vi "Main.vi"() -> ()   [LabVIEW 2020]
doc: "Cet exemple de projet Mesure continue est basé sur le modèle Gestionnaire de messages dans une file d'attente.\n\nLa boucle de gestion d'événements génère des messages en fonction des actions sur l'interface utilisateur.\n\nLa boucle de gestion de messages traite les messages générés par la boucle de gestion d'événements ou par d'autres messages. Il y a aussi des sous-VIs de boucle de gestion de messages d'acquisition et d'enregistrement, ainsi qu'une boucle de mise à jour du graphe déroulant."
uses:
  Settings/Settings.ctl
  Acquisition/Hardware Configuration.ctl
  Acquisition/Signal Type.ctl
  Logging/Logging Configuration.ctl
  controls/UI Data.ctl
  controls/UI State.ctl
  <vilib>/Waveform/WDTOps.llb/WDT Index Channel DBL.vi
  support/Message Queue/Enqueue Message (Single).vi
  support/Message Queue/Enqueue Message (Array).vi
  <vilib>/Utility/error.llb/Error Cluster From Error Code.vi
  <vilib>/ErrorRing/Error Ring.xnode
  Acquisition/Acquisition.lvlib
  Logging/Logging.lvlib
  Settings/Settings.lvlib
  support/User Event - Stop/User Event - Stop.lvlib
  support/Message Queue/Message Queue.lvlib
  Settings/Settings Dialog.vi
panel:
  in  "Panneaux":T1(tab)
  in  "Moyennage sélectionneur":bool
  in  "Choix moyennage":dbl
  in  "Mode longueur d'onde":bool=TRUE
  in  "Sélectionneur de longueur d'onde":dbl=500.0 min=500.0 max=2500.0 step=1.0
  in  "Longueur d'onde":bool
  out "Données":waveform(dbl)[](graph)
  out "État":string
  in  "Quitter":bool
  in  "Arrêter":bool
  in  "Démarrer":bool
  in  "Paramètres":bool
  out "Tableau 2":dbl[](array[numeric])
  # "MAPA Tech"
  # "Automatique"
  # "Manuel"
  # "MAPA Tech"
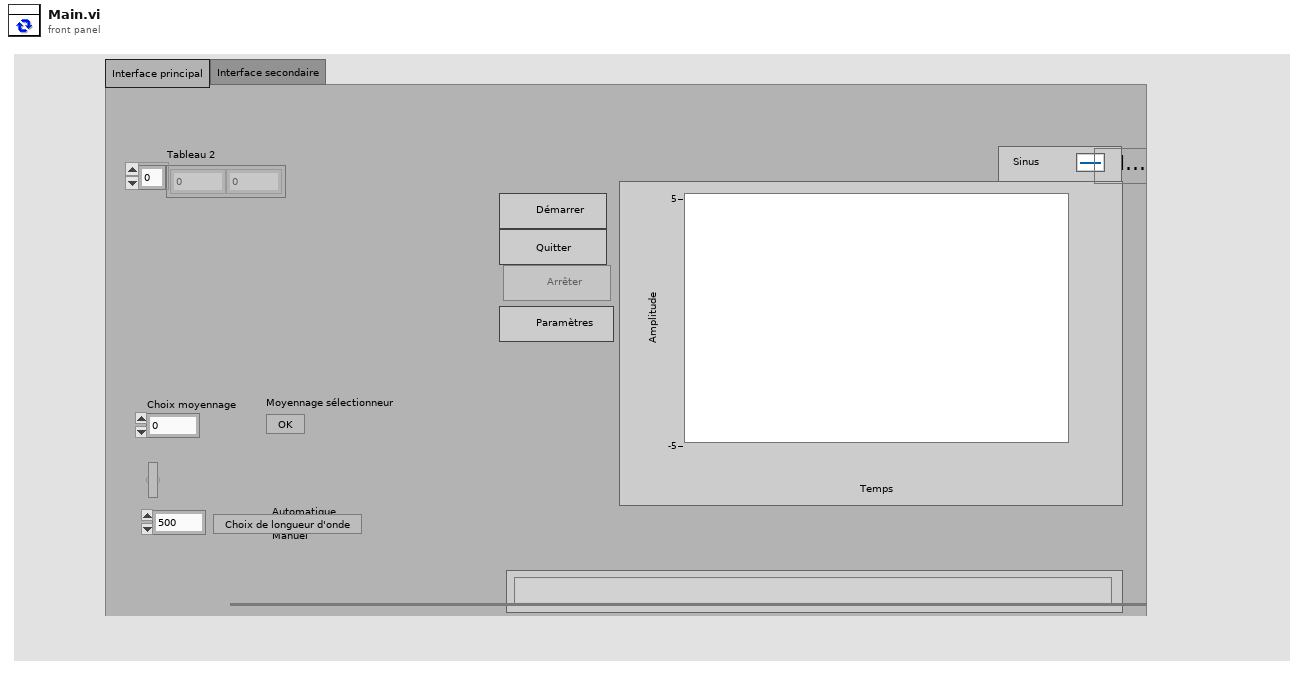
[diagram p1: front panel]
types:
  T1 = enum32{"Interface principal", "Interface secondaire"}
  T2 = typedef "UI State.ctl" = enum16{"Idle", "Acquiring and Logging", "Waiting for Exit", "Waiting for Exit (Acq Stopped)", "Waiting for Exit (Log Stopped)", "Waiting for Stop", "Waiting for Stop (Acq Stopped)", "Waiting for Stop (Log Stopped)"}
  T3 = typedef "UI Data.ctl" = cluster{"Réf. de Démarrer":refnum<vi>, "Réf. d'Arrêter":refnum<vi>, "Réf. de Paramètres":refnum<vi>, "Réf. de Quitter":refnum<vi>, "Réf. d'état":refnum<vi>, "Réf. de données":refnum<vi>, "Ref. longueur d'onde":refnum<vi>, "Ref. Choix mode longueur d'onde":refnum<vi>, "Ref. Moyennage sélectionneur":refnum<vi>}
  T4 = typedef "Settings.lvlib/Settings.ctl" = cluster{"Configuration du matériel":T5, "Configuration de l'enregistrement":T7, "Cluster test":cluster{"Numérique":dbl, "Numérique 2":dbl}}
  T5 = typedef "Acquisition.lvlib/Hardware Configuration.ctl" = cluster{"Refnum de matériel <À remplacer>":string, "Type de signal <À remplacer>":T6}
  T6 = typedef "Acquisition.lvlib/Signal Type.ctl" = enum16{"Sine Wave", "Square with Noise", "Signal triangulaire", "Simulation DAQ"}
  T7 = typedef "Logging.lvlib/Logging Configuration.ctl" = cluster{"Chemin de base du fichier journal":path, "Référence de fichier TDMS":refnum<k34>}
  T8 = cluster{"état":bool, "code":i32, "source":string}
  T9 = typedef "Message Queue.lvlib/All Message Queues.ctl" = cluster{"IU":refnum<queue>, "Acquisition":refnum<queue>, "Enregistrement":refnum<queue>}
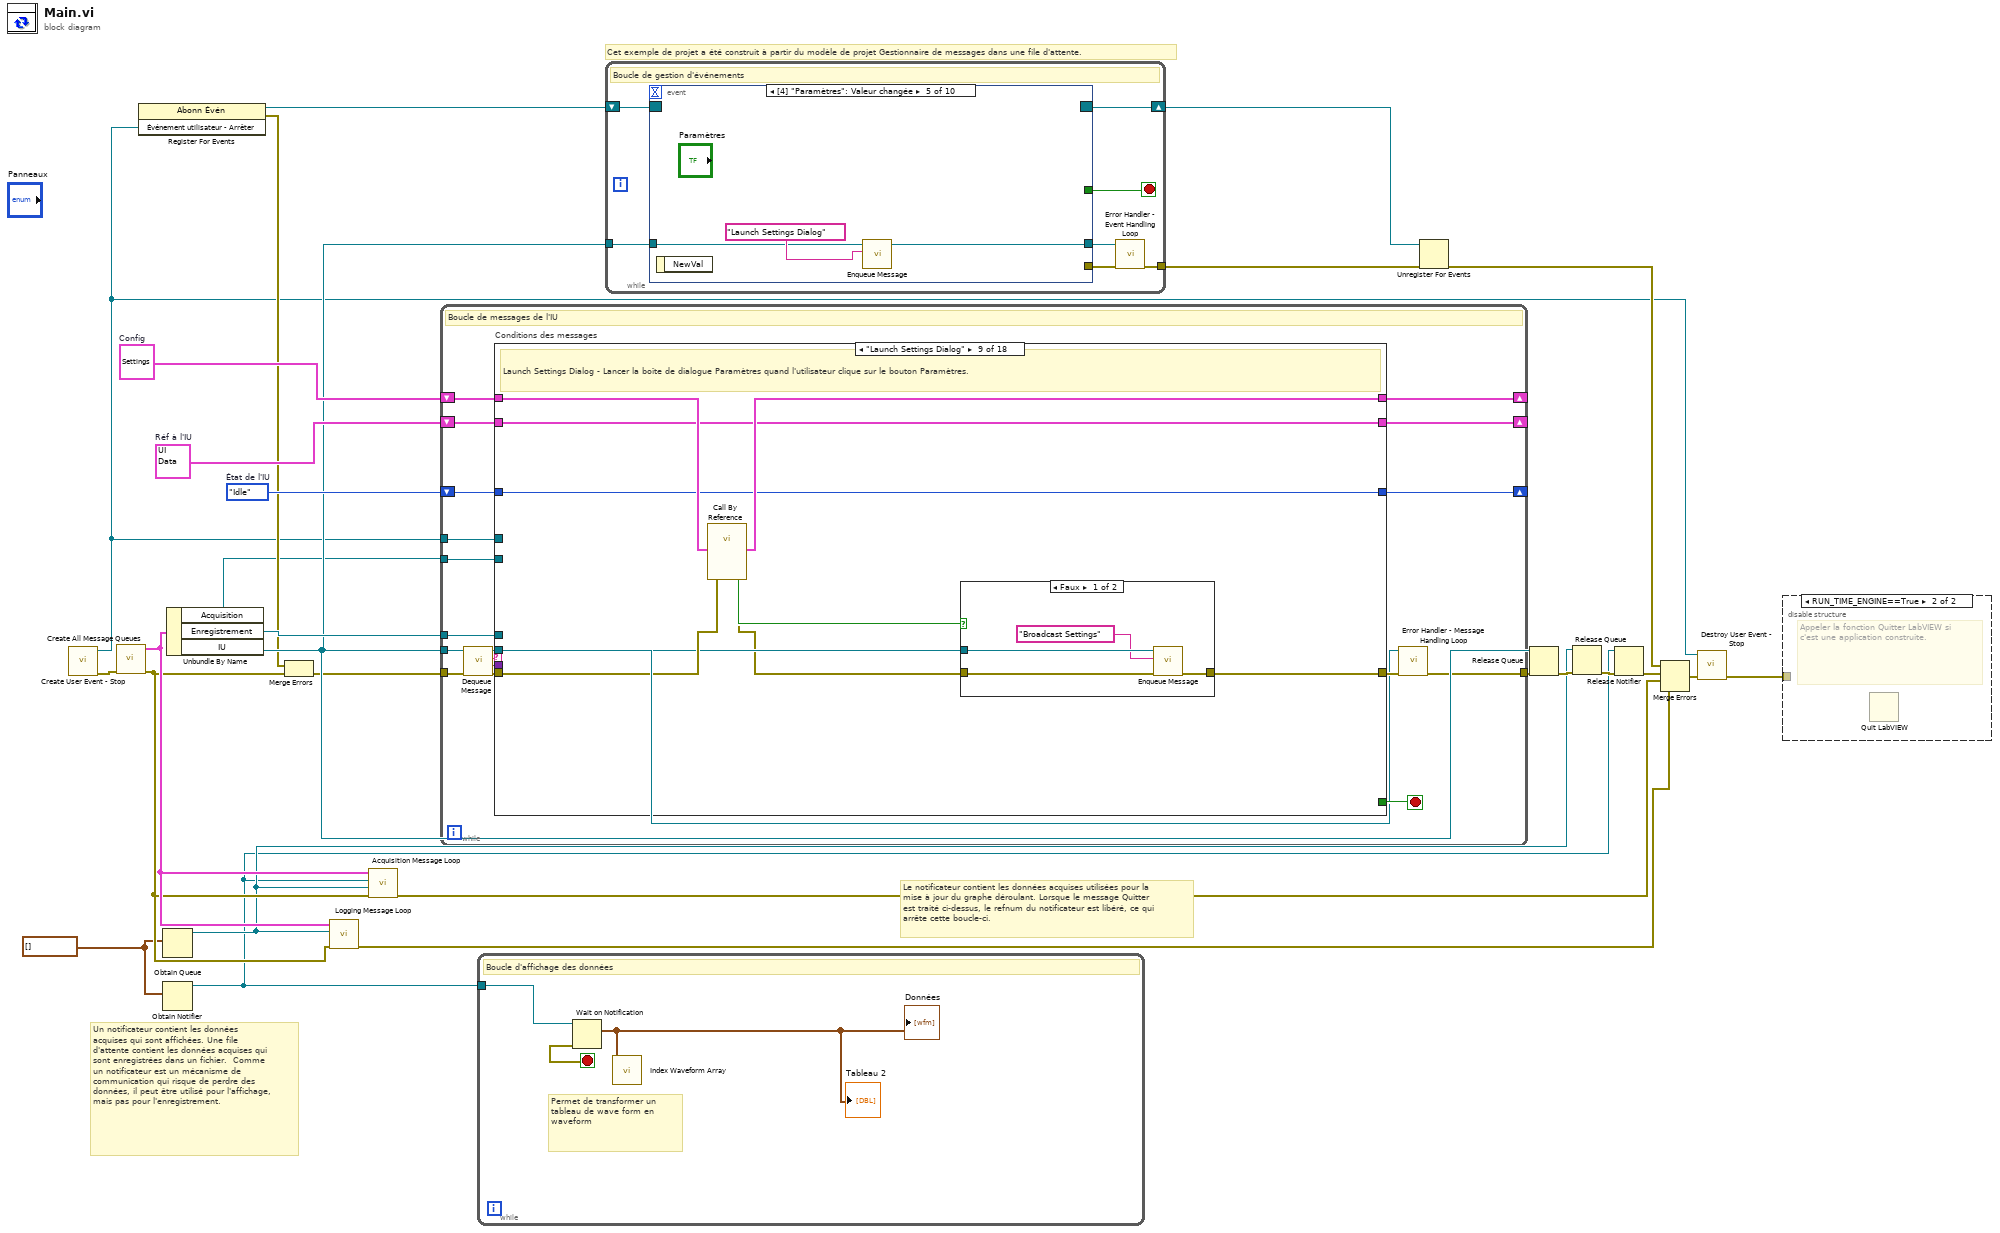
[diagram p0: block diagram]
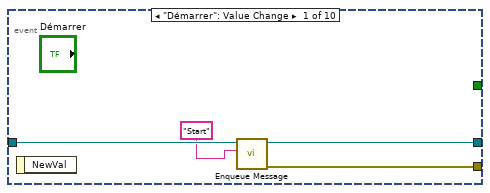
[diagram p3: hidden frame]
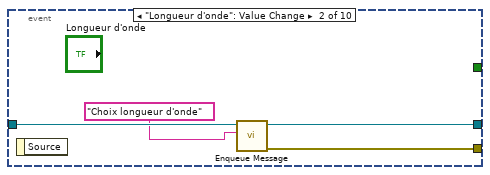
[diagram p4: hidden frame]
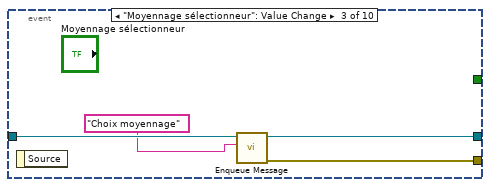
[diagram p5: hidden frame]
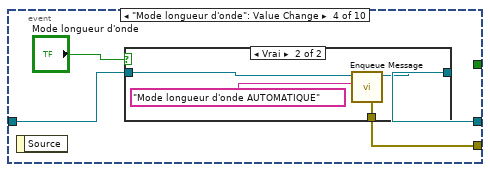
[diagram p6: hidden frame]
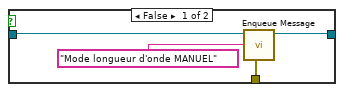
[diagram p7: hidden frame]
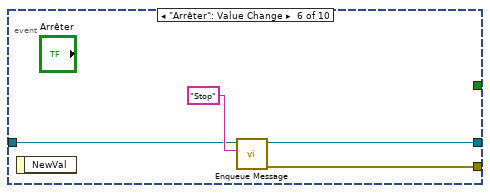
[diagram p8: hidden frame]
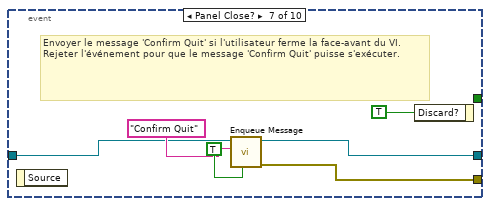
[diagram p9: hidden frame]
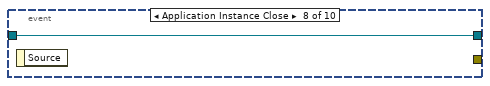
[diagram p10: hidden frame]
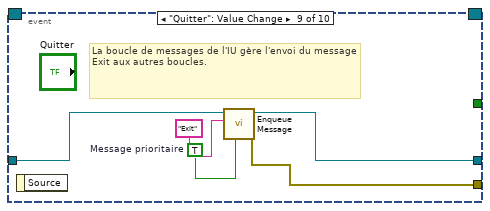
[diagram p11: hidden frame]
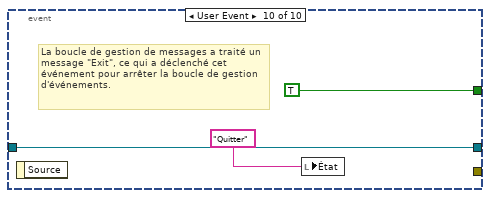
[diagram p12: hidden frame]
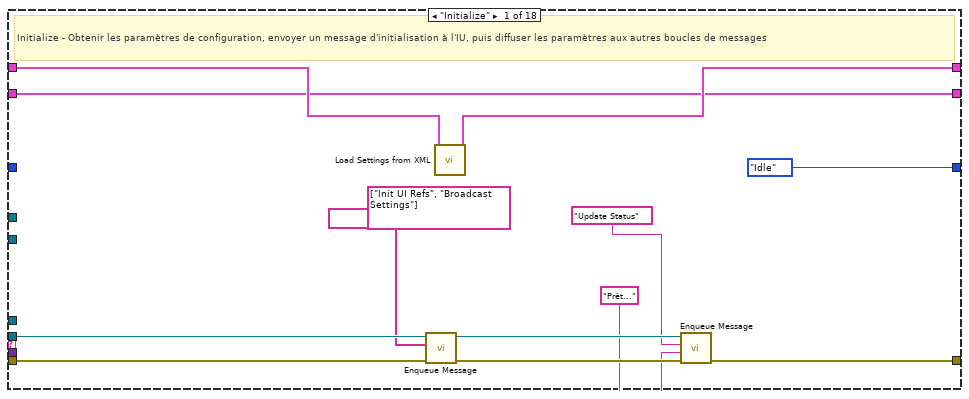
[diagram p13: hidden frame]
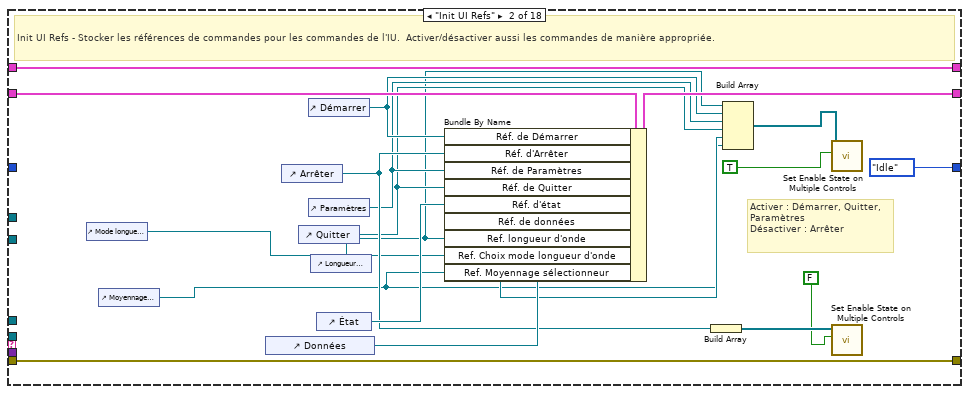
[diagram p14: hidden frame]
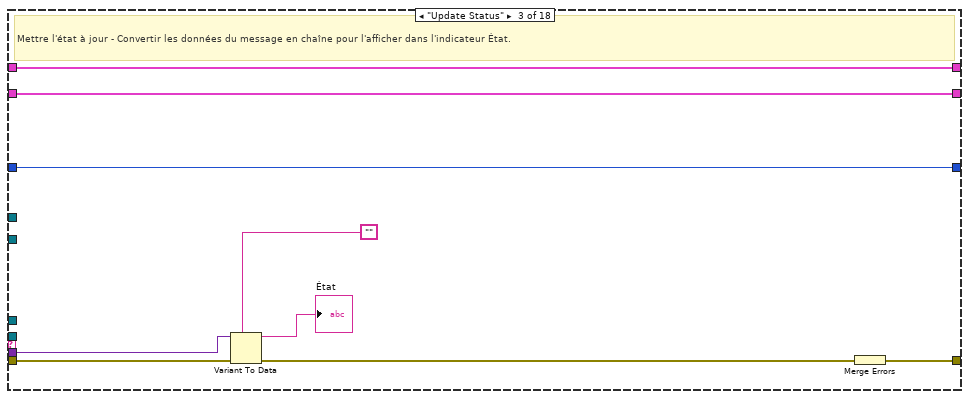
[diagram p15: hidden frame]
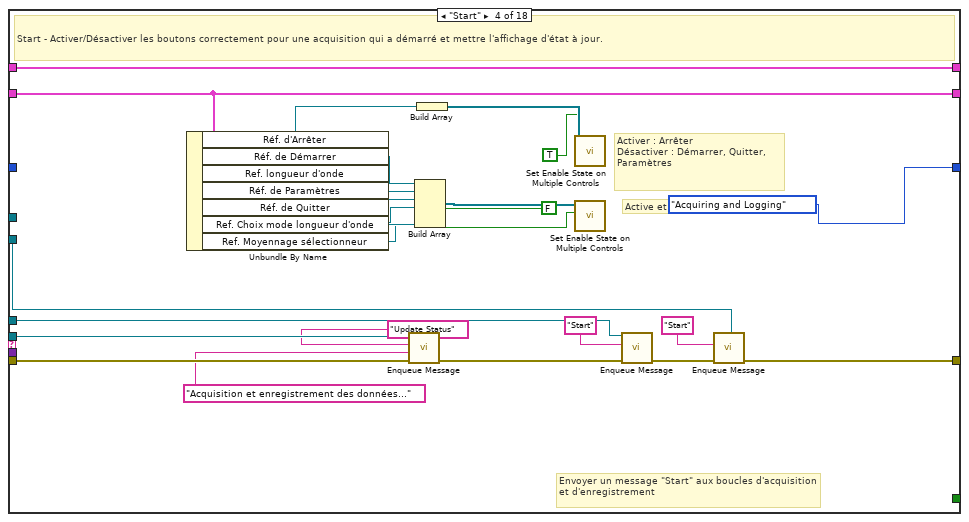
[diagram p16: hidden frame]
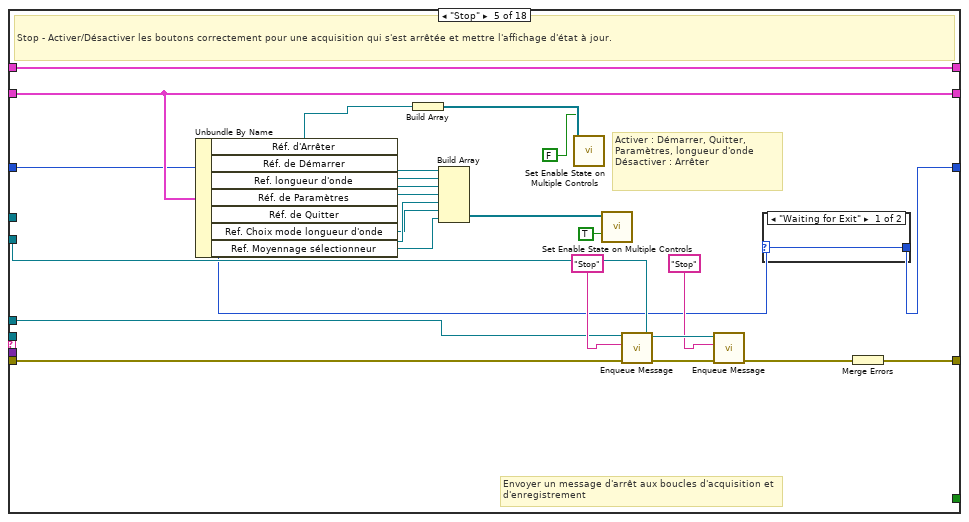
[diagram p17: hidden frame]
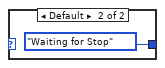
[diagram p18: hidden frame]
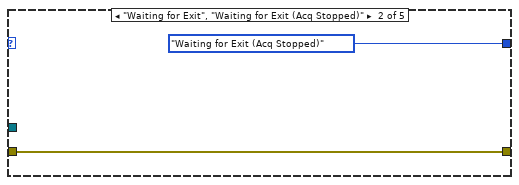
[diagram p20: hidden frame]
diagram:
  w15 = UI_State."Idle"  # État de l'IU
  w1 = waveform(dbl)[] []
  w17 = T3 {"Réf. de Démarrer"=refnum, "Réf. d'Arrêter"=refnum, "Réf. de Paramètres"=refnum, "Réf. de Quitter"=refnum, "Réf. d'état"=refnum, "Réf. de données"=refnum, "Ref. longueur d'onde"=refnum, "Ref. Choix mode longueur d'onde"=refnum, "Ref. Moyennage sélectionneur"=refnum}  # Réf à l'IU
  w20 = T4 {"Configuration du matériel"={"Refnum de matériel <À remplacer>"="", "Type de signal <À remplacer>"=enum."Simulation DAQ"}, "Configuration de l'enregistrement"={"Chemin de base du fichier journal"=path "", "Référence de fichier TDMS"=refnum}, "Cluster test"={"Numérique"=15.0, "Numérique 2"=0.0}}  # Config
  # "Cet exemple de projet a été construit à partir du modèle de projet Gestionnaire de messages dans une file d'attente."
  # "Un notificateur contient les données acquises qui sont affichées. Une file d'attente contient les données acquises qui sont enregistrées dans un fichier.  Comme un notificateur est un mécanisme de communication qui risque de perdre des données, il peut être utilisé pour l'affichage, mais pas pour l'enregistrement."
  # "Le notificateur contient les données acquises utilisées pour la mise à jour du graphe déroulant. Lorsque le message Quitter est traité ci-dessus, le refnum du notificateur est libéré, ce qui arrête cette boucle-ci."
  n1 = call "Create User Event - Stop.vi"() -> ("error out"=w24:T8, "Événement utilisateur - Arrêter"=w2:refnum<user-event>)  [unwired: 10 in]
  n2 = call "Create All Message Queues.vi"("error in (no error)"=w24) -> ("error out"=w21:T8, "Files d'attente de messages en sortie"=w23:T9)  [unwired: 9 in]
  n3 = register-events(w2) -> (reference out=w6:refnum<event-registration>, error out=w4:errorcluster)  [unwired: 2 in]
  n4 = Obtain Queue(element data type=w1) -> (queue out=w8:refnum<queue>)  [unwired: 4 in, 2 out]
  n5 = Obtain Notifier(notification data type=w1) -> (notifier out=w7:refnum<notifier>)  [unwired: 3 in, 2 out]
  n6 = Unbundle By Name(w23) -> ("Acquisition"=w3:refnum<queue>, "Enregistrement"=w16:refnum<queue>, "IU"=w13:refnum<queue>)
  n7 = Merge Errors(w4, w21) -> (w5:errorcluster)
  n8 = call "Logging Message Loop.vi"("error in (no error)"=w21, "File d'attente de données"=w8, "Files d'attente de messages"=w23) -> ("error out"=w22:T8)  [unwired: 8 in]
  n9 = call "Acquisition Message Loop.vi"("error in (no error)"=w21, "File d'attente de données"=w8, "Notificateur de données"=w7, "Files d'attente de messages"=w23) -> ("error out"=w25:T8)  [unwired: 7 in]
  n10 = while {
    tunnel: w13 -> [w39]
    tunnel: w2 -> [w44]
    shift-right: [w38] -> _
    shift-left: w20 -> [w37]
    shift-right: [w35] -> _
    shift-left: w17 -> [w36]
    tunnel: w3 -> [w34]
    tunnel: w16 -> [w33]
    shift-right: [w28] -> _
    shift-left: w15 -> [w29]
    tunnel: w5 -> [w43]
    tunnel: [w32] -> w27
    stop <- w45 stop-if-true
    # "Boucle de messages de l'IU"
    n11 = call "Dequeue Message.vi"("error in (no error)"=w43, "File d'attente de messages"=w39) -> ("error out"=w42:T8, "Données de message"=w40:variant, "Message"=w41:string, "File d'attente de message dup."=w30:refnum<queue>)  [unwired: 6 in]
    n12 = case "Conditions des messages" shown="\"Launch Settings Dialog\"" w41 {
      selector: w41 -> [_ _ _ _ _ _ _ _ _ _ _ _ _ _ _ _ _ w345]
      tunnel: w30 -> [w49 _ _ w109 _ w137 w162 _ w202 _ w223 _ _ w286 w306 w323 w340 _]
      tunnel: w42 -> [w48 w75 w83 w108 w131 w138 w163 w190 w204 w211 w222 w251 w268 w289 w309 w326 w343 _]
      tunnel: [w53 w75 w84 w93 w132 w135 w160 w196 w197 w214 w221 w261 w267 w288 w308 w325 w342 w344] -> w31
      tunnel: [_ _ _ _ _ _ _ _ _ _ _ TRUE _ _ _ _ _ _] -> w45
      tunnel: w40 -> [_ _ w82 _ _ _ _ _ _ w215 _ w249 _ _ _ _ _ _]
      tunnel: w44 -> [_ _ _ _ _ _ _ _ _ _ _ w262 _ _ _ _ _ _]
      tunnel: [w56 w74 w78 w107 w130 w141 w166 w194 w201 w219 w226 w260 w266 w287 w307 w324 w341 w348] -> w38
      tunnel: w37 -> [w57 w74 w78 w107 w130 w141 w166 w194 w205 w219 w226 w260 w266 w287 w307 w324 w341 w348]
      tunnel: w36 -> [w50 w73 w77 w104 w129 w140 w165 w188 w199 w218 w225 w259 w265 w277 w298 w317 w334 w347]
      tunnel: [w50 w70 w77 w104 w129 w140 w165 w188 w199 w218 w225 w259 w265 w277 w298 w317 w334 w347] -> w35
      tunnel: w34 -> [_ _ _ w92 w118 _ _ w187 _ _ _ w258 _ _ _ _ _ _]
      tunnel: w33 -> [_ _ _ w95 w121 _ _ w186 _ _ _ w257 _ _ _ _ _ _]
      tunnel: w29 -> [_ _ w76 _ w115 w139 w164 w185 w198 w213 w224 _ w264 _ _ _ _ w346]
      tunnel: [UI_State."Idle" ("UI State") UI_State."Idle" ("UI State") w76 UI_State."Acquiring and Logging" ("UI State") w116 w136 w161 w185 w198 w213 w220 UI_State."Idle" ("UI State") w264 UI_State."Acquiring and Logging" ("UI State") UI_State."Acquiring and Logging" ("UI State") UI_State."Acquiring and Logging" ("UI State") UI_State."Acquiring and Logging" ("UI State") w346] -> w28
      frame "Initialize" {
        # "Initialize - Obtenir les paramètres de configuration, envoyer un message d'initialisation à l'IU, puis diffuser les paramètres aux autres boucles de messages"
        n13 = call-poly "Enqueue Message.vi"("error in (no error)"=w48, "Tableau de messages"=string[] ["Init UI Refs", "Broadcast Settings"], "File d'attente de messages"=w49) -> ("error out"=w55:T8, "File d'attente de message dup."=w54:refnum<queue>)  [unwired: 7 in]
        n14 = call "Load Settings from XML.vi"("Paramètres en entrée"=w57) -> ("Paramètres en sortie"=w56:T4)  [unwired: 9 in, 1 out]
        n15 = call-poly "Enqueue Message.vi"("error in (no error)"=w55, "Données de message"="Prêt..." ("Ready..."), "Message"="Update Status", "File d'attente de messages"=w54) -> ("error out"=w53:T8)  [unwired: 6 in, 1 out]
      }
      frame "Init UI Refs" {
        # "Activer : Démarrer, Quitter, Paramètres\nDésactiver : Arrêter"
        # "Init UI Refs - Stocker les références de commandes pour les commandes de l'IU.  Activer/désactiver aussi les commandes de manière appropriée."
        n16 = control-ref of="Mode longueur d'onde"() -> (w59:refnum<vi>)
        n17 = control-ref of="Moyennage sélectionneur"() -> (w58:refnum<vi>)
        n18 = control-ref of="Données"() -> (w71:refnum<vi>)
        n19 = control-ref of="Arrêter"() -> (w65:refnum<vi>)
        n20 = control-ref of="Quitter"() -> (w62:refnum<vi>)
        n21 = control-ref of="Démarrer"() -> (w64:refnum<vi>)
        n22 = control-ref of="Paramètres"() -> (w63:refnum<vi>)
        n23 = control-ref of="Longueur d'onde"() -> (w60:refnum<vi>)
        n24 = control-ref of="État"() -> (w72:refnum<vi>)
        n25 = Bundle By Name(cluster=w73, "Réf. de Démarrer"=w64, "Réf. d'Arrêter"=w65, "Réf. de Paramètres"=w63, "Réf. de Quitter"=w62, "Réf. d'état"=w72, "Réf. de données"=w71, "Ref. longueur d'onde"=w60, "Ref. Choix mode longueur d'onde"=w59, "Ref. Moyennage sélectionneur"=w58) -> (w70:T3)
        n26 = Build Array(w65) -> (w67:refnum<vi>[])
        n27 = Build Array(w60, w64, w63, w62, w59, w58) -> (w68:refnum<vi>[])
        n28 = call "Set Enable State on Multiple Controls.vi"("Activé ?"=TRUE ("Enable?"), "Commandes"=w68) -> ()  [unwired: 10 in]
        n29 = call "Set Enable State on Multiple Controls.vi"("Activé ?"=FALSE ("Enable?"), "Commandes"=w67) -> ()  [unwired: 10 in]
      }
      frame "Update Status" {
        # "Mettre l'état à jour - Convertir les données du message en chaîne pour l'afficher dans l'indicateur État."
        n30 = Variant To Data(error in=w83, type="" ("Empty String Constant"), Variant=w82) -> (data=→"État":string, error out=w80:errorcluster)
        n31 = Merge Errors(w80) -> (w84:errorcluster)
      }
      frame "Start" {
        # "Active et désactive les boutons!"
        # "Envoyer un message \"Start\" aux boucles d'acquisition et d'enregistrement"
        # "Activer : Arrêter\nDésactiver : Démarrer, Quitter, Paramètres"
        # "Start - Activer/Désactiver les boutons correctement pour une acquisition qui a démarré et mettre l'affichage d'état à jour."
        n32 = Unbundle By Name(w104) -> ("Réf. d'Arrêter"=w99:refnum<vi>, "Réf. de Démarrer"=w98:refnum<vi>, "Ref. longueur d'onde"=w89:refnum<vi>, "Réf. de Paramètres"=w88:refnum<vi>, "Réf. de Quitter"=w87:refnum<vi>, "Ref. Choix mode longueur d'onde"=w86:refnum<vi>, "Ref. Moyennage sélectionneur"=w85:refnum<vi>)
        n33 = call-poly "Enqueue Message.vi"("error in (no error)"=w108, "Données de message"="Acquisition et enregistrement des données..." ("Acquiring and Logging..."), "Message"="Update Status", "File d'attente de messages"=w109) -> ("error out"=w97:T8)  [unwired: 6 in, 1 out]
        n34 = Build Array(w98, w89, w88, w87, w86, w85) -> (w102:refnum<vi>[])
        n35 = Build Array(w99) -> (w101:refnum<vi>[])
        n36 = call "Set Enable State on Multiple Controls.vi"("Activé ?"=TRUE ("Enable?"), "Commandes"=w101) -> ()  [unwired: 10 in]
        n37 = call "Set Enable State on Multiple Controls.vi"("Activé ?"=FALSE ("Enable?"), "Commandes"=w102) -> ()  [unwired: 10 in]
        n38 = call-poly "Enqueue Message.vi"("error in (no error)"=w97, "Message"="Start", "File d'attente de messages"=w95) -> ("error out"=w94:T8)  [unwired: 7 in, 1 out]
        n39 = call-poly "Enqueue Message.vi"("error in (no error)"=w94, "Message"="Start", "File d'attente de messages"=w92) -> ("error out"=w93:T8)  [unwired: 7 in, 1 out]
      }
      frame "Stop" {
        # "Envoyer un message d'arrêt aux boucles d'acquisition et d'enregistrement"
        # "Activer : Démarrer, Quitter, Paramètres, longueur d'onde\nDésactiver : Arrêter"
        # "Stop - Activer/Désactiver les boutons correctement pour une acquisition qui s'est arrêtée et mettre l'affichage d'état à jour."
        n40 = Unbundle By Name(w129) -> ("Réf. d'Arrêter"=w124:refnum<vi>, "Réf. de Démarrer"=w123:refnum<vi>, "Ref. longueur d'onde"=w114:refnum<vi>, "Réf. de Paramètres"=w113:refnum<vi>, "Réf. de Quitter"=w112:refnum<vi>, "Ref. Choix mode longueur d'onde"=w111:refnum<vi>, "Ref. Moyennage sélectionneur"=w110:refnum<vi>)
        n41 = Build Array(w124) -> (w126:refnum<vi>[])
        n42 = Build Array(w114, w123, w114, w113, w112, w111, w110) -> (w127:refnum<vi>[])
        n43 = call "Set Enable State on Multiple Controls.vi"("Activé ?"=FALSE ("Enable?"), "Commandes"=w126) -> ()  [unwired: 10 in]
        n44 = call "Set Enable State on Multiple Controls.vi"("Activé ?"=TRUE ("Enable?"), "Commandes"=w127) -> ()  [unwired: 10 in]
        n45 = call-poly "Enqueue Message.vi"("error in (no error)"=w131, "Message"="Stop", "File d'attente de messages"=w121) -> ("error out"=w120:T8)  [unwired: 7 in, 1 out]
        n46 = call-poly "Enqueue Message.vi"("error in (no error)"=w120, "Message"="Stop", "File d'attente de messages"=w118) -> ("error out"=w119:T8)  [unwired: 7 in, 1 out]
        n47 = case shown="\"Waiting for Exit\"" w115 {
          selector: w115 -> [w133 _]
          tunnel: [w133 UI_State."Waiting for Stop" ("UI State")] -> w116
          frame "Waiting for Exit" {
          }
          frame Default {
          }
        }
        n48 = Merge Errors(w119) -> (w132:errorcluster)
      }
      frame "Acquisition Stopped" {
        # "Logique déterminant quelle action entreprendre quand l'acquisition s'est arrêtée."
        n49 = case shown="Par défaut" w139 {
          selector: w139 -> [w143 _ _ _ _]
          tunnel: w138 -> [w142 w145 w147 w153 w159]
          tunnel: w137 -> [_ _ _ w151 w156]
          tunnel: [w143 UI_State."Waiting for Exit (Acq Stopped)" ("UI State") UI_State."Waiting for Stop (Acq Stopped)" ("UI State") UI_State."Idle" ("UI State") UI_State."Idle" ("UI State")] -> w136
          tunnel: [w142 w145 w147 w152 w157] -> w135
          frame Default {
          }
          frame "Waiting for Exit", "Waiting for Exit (Acq Stopped)" {
          }
          frame "Waiting for Stop", "Waiting for Stop (Acq Stopped)" {
          }
          frame "Waiting for Exit (Log Stopped)" {
            # "Si nous attendons pour quitter et que l'enregistrement s'est déjà arrêté, le message \"Acquisition Stopped\" indique qu'il est temps de quitter."
            n50 = call-poly "Enqueue Message.vi"("Message prioritaire ? (F)"=TRUE ("Priority Message? (F)"), "error in (no error)"=w153, "Message"="Exit", "File d'attente de messages"=w151) -> ("error out"=w152:T8)  [unwired: 6 in, 1 out]
          }
          frame "Waiting for Stop (Log Stopped)" {
            # "Si nous attendons pour arrêter et que l'enregistrement s'est déjà arrêté, le message \"Acquisition Stopped\" indique qu'il est temps d'arrêter."
            n51 = call-poly "Enqueue Message.vi"("error in (no error)"=w159, "Données de message"="Prêt..." ("Ready..."), "Message"="Update Status", "File d'attente de messages"=w156) -> ("error out"=w157:T8)  [unwired: 6 in, 1 out]
          }
        }
      }
      frame "Logging Stopped" {
        # "Logique déterminant quelle action entreprendre quand l'enregistrement s'est arrêté."
        n52 = case shown="\"Waiting for Stop (Acq Stopped)\"" w164 {
          selector: w164 -> [w168 _ _ _ _]
          tunnel: w163 -> [w167 w170 w172 w178 w181]
          tunnel: w162 -> [_ _ _ w176 w180]
          tunnel: [w168 UI_State."Waiting for Exit (Log Stopped)" ("UI State") UI_State."Waiting for Stop (Log Stopped)" ("UI State") UI_State."Idle" ("UI State") UI_State."Idle" ("UI State")] -> w161
          tunnel: [w167 w170 w172 w177 w179] -> w160
          frame Default {
          }
          frame "Waiting for Exit", "Waiting for Exit (Log Stopped)" {
          }
          frame "Waiting for Stop", "Waiting for Stop (Log Stopped)" {
          }
          frame "Waiting for Exit (Acq Stopped)" {
            # "Si nous attendons pour quitter et que l'acquisition s'est déjà arrêtée, le message \"Logging Stopped\" indique qu'il est temps de quitter."
            n53 = call-poly "Enqueue Message.vi"("Message prioritaire ? (F)"=TRUE ("Priority Message? (F)"), "error in (no error)"=w178, "Message"="Exit", "File d'attente de messages"=w176) -> ("error out"=w177:T8)  [unwired: 6 in, 1 out]
          }
          frame "Waiting for Stop (Acq Stopped)" {
            # "Si nous attendons pour arrêter et que l'acquisition s'est déjà arrêtée, le message \"Logging Stopped\" indique qu'il est temps d'arrêter."
            n54 = call-poly "Enqueue Message.vi"("error in (no error)"=w181, "Données de message"="Prêt..." ("Ready..."), "Message"="Update Status", "File d'attente de messages"=w180) -> ("error out"=w179:T8)  [unwired: 6 in, 1 out]
          }
        }
      }
      frame "Broadcast settings" {
        w189 = "Update Settings" ("Message")
        # "Broadcast settings - Envoyer le message 'Update Settings' aux boucles de messages d'enregistrement et d'acquisition."
        n55 = Unbundle By Name(w194) -> ("Configuration du matériel"=w193:T5, "Configuration de l'enregistrement"=w192:T7)
        n56 = call-poly "Enqueue Message.vi"("Données de message"=w193, "Message"=w189, "File d'attente de messages"=w187) -> ("error out"=w195:T8)  [unwired: 7 in, 1 out]
        n57 = call-poly "Enqueue Message.vi"("error in (no error)"=w195, "Données de message"=w192, "Message"=w189, "File d'attente de messages"=w186) -> ("error out"=w191:T8)  [unwired: 6 in, 1 out]
        n58 = Merge Errors(w191, w190) -> (w196:errorcluster)
      }
      frame "Launch Settings Dialog" {
        # "Launch Settings Dialog - Lancer la boîte de dialogue Paramètres quand l'utilisateur clique sur le bouton Paramètres."
        n59 = call-by-ref "?"("error in (no error)"=w204, "Paramètres en entrée"=w205) -> ("error out"=w200:T8, "Annulation ?"=w203:bool, "Paramètres en sortie"=w201:T4)  [unwired: 8 in, 3 out]
        n60 = case shown="Faux" w203 {
          tunnel: w202 -> [w209 _]
          tunnel: w200 -> [w208 w210]
          tunnel: [w207 w210] -> w197
          frame False {
            n61 = call-poly "Enqueue Message.vi"("error in (no error)"=w208, "Message"="Broadcast Settings", "File d'attente de messages"=w209) -> ("error out"=w207:T8)  [unwired: 7 in, 1 out]
          }
          frame True {
          }
        }
      }
      frame "Error" {
        # "Error - Afficher une boîte de dialogue d'erreur. Ce message est envoyé par les VIs \"Error Handler\" à la fin de l'exécution de chaque boucle de cette application."
        n62 = Variant To Data(error in=w211, type=errorcluster {"status"=FALSE, "code"=0, "source"=""} ("error constant"), Variant=w215) -> (data=w212:errorcluster, error out=w216:errorcluster)
        n63 = call <vilib>:"Simple Error Handler.vi"("error in (no error)"=w212) -> ()  [unwired: 4 in, 5 out]
        n64 = Merge Errors(w216) -> (w214:errorcluster)
      }
      frame "Confirm Quit" {
        # "Confirm Quit - Message qui confirme si l'utilisateur voulait vraiment quitter l'application."
        n65 = case shown="\"Acquiring and Logging\"" w224 {
          tunnel: w223 -> [w232 w236]
          tunnel: w222 -> [w231 w235]
          tunnel: [w230 w234] -> w221
          tunnel: [UI_State."Idle" ("UI State") w233] -> w220
          frame Default {
            # "Si 'Confirm Quit' survient alors que le système est inactif, le message de confirmation est inutile."
            n66 = call-poly "Enqueue Message.vi"("Message prioritaire ? (F)"=TRUE ("Priority Message? (F)"), "error in (no error)"=w231, "Message"="Exit", "File d'attente de messages"=w232) -> ("error out"=w230:T8)  [unwired: 6 in, 1 out]
          }
          frame "Acquiring and Logging" {
            n67 = Two Button Dialog(message="Voulez-vous vraiment quitter en cours d'acquisition ?" ("Confirm Quit Message"), 1:"Non" ("No"), 2:"Oui" ("Yes")) -> (T button?=w237:bool)
            n68 = case shown="Vrai" w237 {
              tunnel: w236 -> [_ w246]
              tunnel: w235 -> [w242 w247]
              tunnel: [w242 w245] -> w234
              tunnel: [UI_State."Acquiring and Logging" ("UI State") UI_State."Waiting for Exit" ("UI State")] -> w233
              frame False {
                # "L'utilisateur ne voulait pas quitter."
              }
              frame True {
                n69 = call-poly "Enqueue Message.vi"("error in (no error)"=w247, "Message"="Stop", "File d'attente de messages"=w246) -> ("error out"=w245:T8)  [unwired: 7 in, 1 out]
              }
            }
          }
        }
      }
      frame "Exit" {
        w253 = TRUE ("Priority Message? (F)")
        w254 = "Exit" ("Message")
        # "Afficher une boîte de dialogue d'erreur si 'Exit' a été appelé suite à une erreur."
        # "Arrêter le VI"
        # "Exit - Envoyer des messages Exit aux boucles d'acquisition et d'enregistrerment, et déclencher l'événement utilisateur pour arrêter la boucle de gestion d'événements."
        n70 = Variant To Data(type=errorcluster {"status"=FALSE, "code"=0, "source"=""} ("error constant"), Variant=w249) -> (data=w248:errorcluster)  [unwired: 1 in, 1 out]
        n71 = call <vilib>:"Simple Error Handler.vi"("error in (no error)"=w248) -> ()  [unwired: 4 in, 5 out]
        n72 = call-poly "Enqueue Message.vi"("Message prioritaire ? (F)"=w253, "error in (no error)"=w251, "Message"=w254, "File d'attente de messages"=w258) -> ("error out"=w255:T8)  [unwired: 6 in, 1 out]
        n73 = call-poly "Enqueue Message.vi"("Message prioritaire ? (F)"=w253, "error in (no error)"=w255, "Message"=w254, "File d'attente de messages"=w257) -> ("error out"=w252:T8)  [unwired: 6 in, 1 out]
        n74 = call "Fire User Event - Stop.vi"("error in (no error)"=w252, "Événement utilisateur - Arrêt"=w262) -> ("error out"=w261:T8)  [unwired: 9 in]
      }
      frame "---Copy This Frame---" {
        # "Dupliquez cette étape pour créer de nouveaux messages.  Changez ce commentaire dans l'étape dupliquée pour décrire ce message."
        n75 = Merge Errors(w268) -> (w267:errorcluster)
      }
      frame "Choix longueur d'onde" {
        # "Activer : \nDésactiver :"
        # "Affiche la longueur d'onde en live.\nComment je fais pour limiter le range\ncomment je fais pour afficher pas en live\ngestion d'erreur?"
        # "Dupliquez cette étape pour créer de nouveaux messages.  Changez ce commentaire dans l'étape dupliquée pour décrire ce message."
        n76 = Unbundle By Name(w277) -> ("Ref. longueur d'onde"=w274:refnum<vi>, "Réf. d'Arrêter"=w272:refnum<vi>, "Réf. de Démarrer"=w271:refnum<vi>, "Réf. de Quitter"=w275:refnum<vi>, "Réf. de Paramètres"=w273:refnum<vi>)
        n77 = Build Array(w271, w275, w274, w273) -> (w279:refnum<vi>[])
        n78 = Build Array(w272) -> (w270:refnum<vi>[])
        n79 = call "Set Enable State on Multiple Controls.vi"("Activé ?"=TRUE ("Enable?"), "Commandes"=w279) -> ()  [unwired: 10 in]
        n80 = Number To Decimal String(number="Sélectionneur de longueur d'onde") -> (decimal integer string=w283:string)  [unwired: 1 in]
        n81 = Concatenate Strings ("Concaténer des chaînes")("La longueur d'onde sélectionné est de ", w283, " nm.") -> (w280:string)
        n82 = call "Set Enable State on Multiple Controls.vi"("Activé ?"=FALSE ("Enable?"), "Commandes"=w270) -> ()  [unwired: 10 in]
        n83 = call-poly "Enqueue Message.vi"("Données de message"=w280, "Message"="Update Status", "File d'attente de messages"=w286) -> ()  [unwired: 7 in, 2 out]
        n84 = Merge Errors(w289) -> (w288:errorcluster)
      }
      frame "Choix moyennage" {
        # "Activer : \nDésactiver :"
        # "Affiche la longueur d'onde en live.\nComment je fais pour limiter le range\ncomment je fais pour afficher pas en live\ngestion d'erreur?"
        # "Dupliquez cette étape pour créer de nouveaux messages.  Changez ce commentaire dans l'étape dupliquée pour décrire ce message."
        n85 = Unbundle By Name(w298) -> ("Réf. d'Arrêter"=w292:refnum<vi>, "Réf. de Démarrer"=w291:refnum<vi>, "Réf. de Quitter"=w296:refnum<vi>, "Réf. de Paramètres"=w290:refnum<vi>)
        n86 = Build Array(w291, w296, w290) -> (w300:refnum<vi>[])
        n87 = Build Array(w292) -> (w294:refnum<vi>[])
        n88 = call "Set Enable State on Multiple Controls.vi"("Activé ?"=TRUE ("Enable?"), "Commandes"=w300) -> ()  [unwired: 10 in]
        n89 = Number To Decimal String(number="Choix moyennage") -> (decimal integer string=w304:string)  [unwired: 1 in]
        n90 = call "Set Enable State on Multiple Controls.vi"("Activé ?"=FALSE ("Enable?"), "Commandes"=w294) -> ()  [unwired: 10 in]
        n91 = Concatenate Strings ("Concaténer des chaînes")("Le moyennage sélectionné est de ", w304, " Hz.") -> (w301:string)
        n92 = call-poly "Enqueue Message.vi"("Données de message"=w301, "Message"="Update Status", "File d'attente de messages"=w306) -> ()  [unwired: 7 in, 2 out]
        n93 = Merge Errors(w309) -> (w308:errorcluster)
      }
      frame "Mode longueur d'onde AUTOMATIQUE" {
        # "Activer : \nDésactiver :"
        # "Dupliquez cette étape pour créer de nouveaux messages.  Changez ce commentaire dans l'étape dupliquée pour décrire ce message."
        n94 = Unbundle By Name(w317) -> ("Ref. longueur d'onde"=w314:refnum<vi>, "Réf. d'Arrêter"=w312:refnum<vi>, "Réf. de Démarrer"=w311:refnum<vi>, "Réf. de Quitter"=w315:refnum<vi>, "Réf. de Paramètres"=w310:refnum<vi>)
        n95 = Build Array(w311, w315, w310) -> (w319:refnum<vi>[])
        n96 = Build Array(w312, w314) -> (w320:refnum<vi>[])
        n97 = call "Set Enable State on Multiple Controls.vi"("Activé ?"=TRUE ("Enable?"), "Commandes"=w319) -> ()  [unwired: 10 in]
        n98 = call "Set Enable State on Multiple Controls.vi"("Activé ?"=FALSE ("Enable?"), "Commandes"=w320) -> ()  [unwired: 10 in]
        n99 = call-poly "Enqueue Message.vi"("Données de message"="Le mode sélectionné pour la longueur d'onde est automatique.", "Message"="Update Status", "File d'attente de messages"=w323) -> ()  [unwired: 7 in, 2 out]
        n100 = Merge Errors(w326) -> (w325:errorcluster)
      }
      frame "Mode longueur d'onde MANUEL" {
        # "Activer : \nDésactiver :"
        # "Affiche la longueur d'onde en live.\nComment je fais pour limiter le range\ncomment je fais pour afficher pas en live\ngestion d'erreur?"
        # "Dupliquez cette étape pour créer de nouveaux messages.  Changez ce commentaire dans l'étape dupliquée pour décrire ce message."
        n101 = Unbundle By Name(w334) -> ("Ref. longueur d'onde"=w330:refnum<vi>, "Réf. d'Arrêter"=w329:refnum<vi>, "Réf. de Démarrer"=w328:refnum<vi>, "Réf. de Quitter"=w332:refnum<vi>, "Réf. de Paramètres"=w327:refnum<vi>)
        n102 = Build Array(w327, w328, w332, w330) -> (w336:refnum<vi>[])
        n103 = Build Array(w329) -> (w337:refnum<vi>[])
        n104 = call "Set Enable State on Multiple Controls.vi"("Activé ?"=TRUE ("Enable?"), "Commandes"=w336) -> ()  [unwired: 10 in]
        n105 = call "Set Enable State on Multiple Controls.vi"("Activé ?"=FALSE ("Enable?"), "Commandes"=w337) -> ()  [unwired: 10 in]
        n106 = call-poly "Enqueue Message.vi"("Données de message"="Le mode sélectionné pour la longueur d'onde est manuel.", "Message"="Update Status", "File d'attente de messages"=w340) -> ()  [unwired: 7 in, 2 out]
        n107 = Merge Errors(w343) -> (w342:errorcluster)
      }
      frame Default {
        # "La condition 'Par défaut' ne s'exécute que s'il y a un message qui n'est défini dans aucune des autres conditions.  Renvoyer une erreur de programmation."
        n108 = xnode ("Error Ring")("paramètre 0"=w345) -> ("sortie d'erreur"=w344:errorcluster)
      }
    }
    n109 = call "Error Handler - Message Handling Loop.vi"("error in (no error)"=w31, "File d'attente de messages"=w30) -> ("erreur en entrée dup."=w32:T8)  [unwired: 8 in, 1 out]
  }
  n110 = while "Data Display Loop" {
    tunnel: w7 -> [w357]
    stop <- w358 stop-if-true
    # "Permet de transformer un tableau de wave form en\nwaveform"
    # "Boucle d'affichage des données"
    n111 = Wait on Notification(notifier=w357) -> (notification=w356:waveform(dbl)[], error out=w358:errorcluster)  [unwired: 3 in, 2 out]
    "Données" <- w356
    "Tableau 2" <- w356
    n112 = call-poly <vilib>:"Index Waveform Array.vi"("waveform array"=w356) -> ()  [unwired: 9 in, 2 out]
  }
  n113 = while {
    tunnel: w13 -> [w364]
    tunnel: [w361] -> w26
    shift-right: [w363] -> w18
    shift-left: w6 -> [w365]
    stop <- w362 stop-if-true
    # "Boucle de gestion d'événements"
    n114 = event shown="[4] \"Paramètres\": Valeur changée" {
      selector: w365 -> [_ _ _ _ _ _ _ _ _ _]
      dyn-events: [_ _ _ _ _ _ _ _ _ _] -> w363
      timeout: _ -> [_ _ _ _ _ _ _ _ _ _]
      tunnel: [_ _ _ _ _ _ _ _ _ TRUE ("Discard?")] -> w362
      tunnel: w364 -> [w369 w373 w377 w380 w391 w395 w400 w403 w405 w409]
      tunnel: [w367 w371 w375 w379 _ w394 w398 _ w408 _] -> w360
      tunnel: [w366 w370 w374 w378 w390 w393 w399 w403 w404 w409] -> w359
      event "Démarrer": Value Change {
        n115 = event-data() -> ()  [unwired: 1 in, 1 out]
        n116 = call-poly "Enqueue Message.vi"("Message"="Start", "File d'attente de messages"=w369) -> ("error out"=w367:T8, "File d'attente de message dup."=w366:refnum<queue>)  [unwired: 8 in]
      }
      event "Longueur d'onde": Value Change {
        n117 = event-data() -> ()  [unwired: 1 in, 1 out]
        n118 = call-poly "Enqueue Message.vi"("Message"="Choix longueur d'onde", "File d'attente de messages"=w373) -> ("error out"=w371:T8, "File d'attente de message dup."=w370:refnum<queue>)  [unwired: 8 in]
      }
      event "Moyennage sélectionneur": Value Change {
        n119 = event-data() -> ()  [unwired: 1 in, 1 out]
        n120 = call-poly "Enqueue Message.vi"("Message"="Choix moyennage", "File d'attente de messages"=w377) -> ("error out"=w375:T8, "File d'attente de message dup."=w374:refnum<queue>)  [unwired: 8 in]
      }
      event "Mode longueur d'onde": Value Change {
        n121 = event-data() -> ()  [unwired: 1 in, 1 out]
        n122 = case shown="Vrai" "Mode longueur d'onde" {
          tunnel: w380 -> [w384 w389]
          tunnel: [w382 w388] -> w379
          tunnel: [w383 w387] -> w378
          frame False {
            n123 = call-poly "Enqueue Message.vi"("Message"="Mode longueur d'onde MANUEL", "File d'attente de messages"=w384) -> ("error out"=w382:T8, "File d'attente de message dup."=w383:refnum<queue>)  [unwired: 8 in]
          }
          frame True {
            n124 = call-poly "Enqueue Message.vi"("Message"="Mode longueur d'onde AUTOMATIQUE", "File d'attente de messages"=w389) -> ("error out"=w388:T8, "File d'attente de message dup."=w387:refnum<queue>)  [unwired: 8 in]
          }
        }
      }
      event "Paramètres": Value Change {
        n125 = event-data() -> ()  [unwired: 1 in, 1 out]
        n126 = call-poly "Enqueue Message.vi"("Message"="Launch Settings Dialog", "File d'attente de messages"=w391) -> ("File d'attente de message dup."=w390:refnum<queue>)  [unwired: 8 in, 1 out]
      }
      event "Arrêter": Value Change {
        n127 = event-data() -> ()  [unwired: 1 in, 1 out]
        n128 = call-poly "Enqueue Message.vi"("Message"="Stop", "File d'attente de messages"=w395) -> ("error out"=w394:T8, "File d'attente de message dup."=w393:refnum<queue>)  [unwired: 8 in]
      }
      event Panel Close? {
        # "Envoyer le message 'Confirm Quit' si l'utilisateur ferme la face-avant du VI. Rejeter l'événement pour que le message 'Confirm Quit' puisse s'exécuter."
        n129 = event-data() -> ()  [unwired: 1 in, 1 out]
        n130 = call-poly "Enqueue Message.vi"("Message prioritaire ? (F)"=TRUE ("Priority Message? (F)"), "Message"="Confirm Quit", "File d'attente de messages"=w400) -> ("error out"=w398:T8, "File d'attente de message dup."=w399:refnum<queue>)  [unwired: 7 in]
        n131 = event-data ("Event Filter Node")("Discard?"=TRUE) -> ()  [unwired: 1 in, 1 out]
      }
      event Application Instance Close {
        n132 = event-data() -> ()  [unwired: 1 in, 1 out]
      }
      event "Quitter": Value Change {
        w406 = TRUE  # Message prioritaire
        # "La boucle de messages de l'IU gère l'envoi du message Exit aux autres boucles."
        n133 = event-data() -> ()  [unwired: 1 in, 1 out]
        n134 = call-poly "Enqueue Message.vi"("Message prioritaire ? (F)"=w406, "Message"="Exit", "File d'attente de messages"=w405) -> ("error out"=w408:T8, "File d'attente de message dup."=w404:refnum<queue>)  [unwired: 7 in]
      }
      event User Event {
        # "La boucle de gestion de messages a traité un message \"Exit\", ce qui a déclenché cet événement pour arrêter la boucle de gestion d'événements."
        n135 = event-data() -> ()  [unwired: 1 in, 1 out]
        n136 = local write "État"("Quitter" ("Exit String")) -> ()
      }
    }
    n137 = call "Error Handler - Event Handling Loop.vi"("error in (no error)"=w360, "File d'attente de messages"=w359) -> ("erreur en entrée dup."=w361:T8)  [unwired: 8 in, 1 out]
  }
  n138 = Unregister For Events(event registration refnum=w18, error in=w26) -> (error out=w19:errorcluster)
  n139 = Release Queue(queue=w13, error in (no error)=w27) -> (error out=w11:errorcluster)  [unwired: 1 in, 2 out]
  n140 = Release Queue(queue=w8, error in (no error)=w11) -> (error out=w10:errorcluster)  [unwired: 1 in, 2 out]
  n141 = Release Notifier(notifier=w7, error in (no error)=w10) -> (error out=w9:errorcluster)  [unwired: 1 in, 2 out]
  n142 = Merge Errors(w19, w9, w25, w22) -> (w14:errorcluster)
  n143 = call "Destroy User Event - Stop.vi"("error in (no error)"=w14, "Événement utilisateur - Arrêt"=w2) -> ("error out"=w12:T8)  [unwired: 9 in]
  n144 = disable-structure "Conditional Disable Structure" shown="RUN_TIME_ENGINE==True" {
    disable-tunnel: w12 -> [_ _]
    frame condition #0 (active) {
    }
    frame condition #1 {
      # "Appeler la fonction Quitter LabVIEW si c'est une application construite."
      n145 = Quit LabVIEW() -> ()  [unwired: 1 in]
    }
  }
